vi "Pad String.vi"(5 "Expected Length":u8, 7 "Pad Character":u8, 8 "error in (no error)":errorcluster, 10 "String To Pad":string, 11 "Listener in":refnum<class "Listener.lvclass">) -> (0 "error out":errorcluster, 2 "Padded String":string, 3 "Listener out":refnum<class "Listener.lvclass">)   [LabVIEW 2019, in "Listener.lvclass"]
uses:
  Listener.lvclass
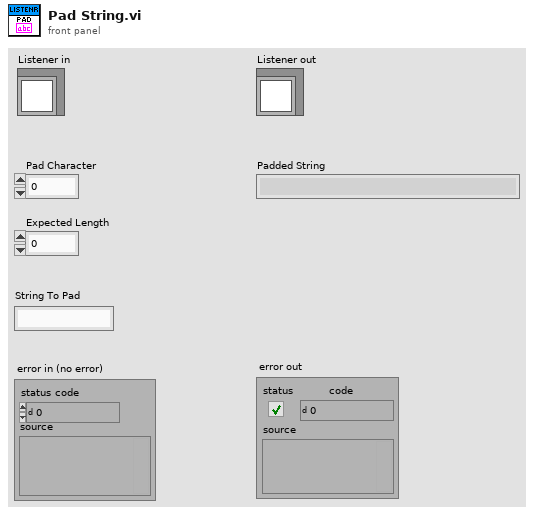
[diagram p1: front panel]
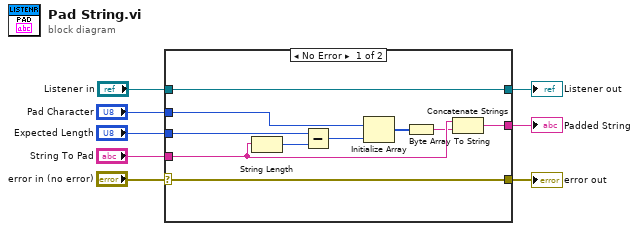
[diagram p0: block diagram]
diagram:
  n1 = case shown="No Error" "error in (no error)" {
    selector: "error in (no error)" -> [w10 w21]
    tunnel: [w18 w20] -> w8
    tunnel: "String To Pad" -> [w17 w20]
    tunnel: "Pad Character" -> [w16 _]
    tunnel: "Expected Length" -> [w15 _]
    tunnel: [w10 w21] -> w4
    tunnel: "Listener in" -> [w9 w19]
    tunnel: [w9 w19] -> w1
    frame No Error {
      n2 = String Length(string=w17) -> (length=w11:i32)
      n3 = Subtract(x=w15, y=w11) -> (x-y=w12:i32)
      n4 = Initialize Array(w16, w12) -> (w14:u8[])
      n5 = Byte Array To String(unsigned byte array=w14) -> (string=w13:string)
      n6 = Concatenate Strings(w17, w13) -> (w18:string)
    }
    frame Error {
    }
  }
  "Padded String" <- w8
  "error out" <- w4
  "Listener out" <- w1
